vi "Copy Template Cases.vi"(7 "Template Case Count":i32=2, 8 "error in (no error)":errorcluster, 9 "Names":string[](array[string]), 10 "Source Templates":i32[](array[numeric]), 11 "Case":refnum<vi>) -> (0 "error out":errorcluster, 2 "Frames":refnum<vi>[](array[refnum]))   [LabVIEW 2020, in "LV-Protoc.lvlib"]
uses:
  LV-Protoc.lvlib
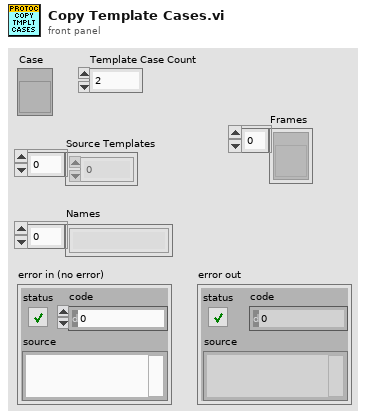
[diagram p1: front panel]
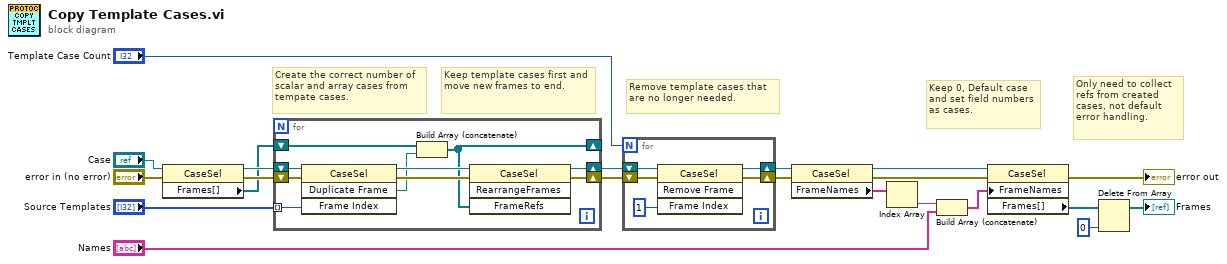
[diagram p0: block diagram]
diagram:
  # "Keep template cases first and move new frames to end."
  # "Only need to collect refs from created cases, not default error handling."
  # "Keep 0, Default case and set field numbers as cases."
  # "Remove template cases that are no longer needed."
  # "Create the correct number of scalar and array cases from tempate cases."
  n1 = property class="CaseSel"(reference="Case", error in="error in (no error)") -> (reference out=w3:refnum<vi>, error out=w4:errorcluster, "Frames[]"=w1:refnum<vi>[])
  n2 = for {
    shift-right: [w23] -> w15
    shift-left: w3 -> [w31]
    shift-right: [w22] -> w14
    shift-left: w4 -> [w30]
    tunnel: "Source Templates" -> [w29] mode=indexing
    shift-right: [w24] -> _
    shift-left: w1 -> [w26]
    n3 = invoke class="CaseSel" method="Duplicate Frame"(reference=w31, error in=w30, "Frame Index"=w29) -> (reference out=w28:refnum<vi>, error out=w27:errorcluster, "Duplicate Frame"=w25:refnum<vi>)  [unwired: 1 in, 1 out]
    n4 = Build Array (concatenate)(w26, w25) -> (w24:refnum<vi>[])
    n5 = invoke class="CaseSel" method="RearrangeFrames"(reference=w28, error in=w27, "FrameRefs"=w24) -> (reference out=w23:refnum<vi>, error out=w22:errorcluster)  [unwired: 1 in, 2 out]
  }
  n6 = for {
    N: "Template Case Count" -> [_]
    shift-right: [w35] -> w13
    shift-left: w15 -> [w36]
    shift-right: [w34] -> w12
    shift-left: w14 -> [w33]
    n7 = invoke class="CaseSel" method="Remove Frame"(reference=w36, error in=w33, "Frame Index"=u32 1) -> (reference out=w35:refnum<vi>, error out=w34:errorcluster)  [unwired: 1 in, 2 out]
  }
  n8 = property class="CaseSel"(reference=w13, error in=w12) -> (reference out=w18:refnum<vi>, error out=w21:errorcluster, "FrameNames"=w20:string[])
  n9 = Index Array(array=w20) -> (element=w19:string)  [unwired: 1 in]
  n10 = Build Array (concatenate)(w19, "Names") -> (w17:string[])
  n11 = property class="CaseSel"(reference=w18, error in=w21, "FrameNames"=w17) -> (error out=→"error out":errorcluster, "Frames[]"=w9:refnum<vi>[])  [unwired: 1 out]
  n12 = Delete From Array(array=w9, index=0) -> (array with subset deleted=→"Frames":refnum<vi>[])  [unwired: 1 in, 1 out]
